vi "PH_uOPA_DelayController.contents.vi"   [LabVIEW 2014, in "PH_uOPA_DelayController.lvlib"]
doc: "This class is forseen to collect andf indicate the measured laser backreflection data.\n\nThis class is part of the PHELIX device layer."
uses:
  PH_uOPA_DelayController.lvlib
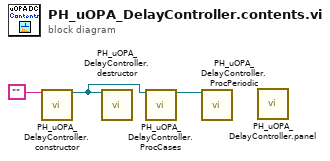
[diagram p0: block diagram]
diagram:
  n1 = call "PH_uOPA_DelayController.constructor.vi"("name"="") -> ("i ref out"=w1:refnum<vi>)  [unwired: 16 in, 2 out]
  n2 = call "PH_uOPA_DelayController.destructor.vi"("i ref in"=w1) -> ()  [unwired: 18 in, 1 out]
  n3 = call "PH_uOPA_DelayController.ProcCases.vi"("i ref in"=w1) -> ("i ref out"=w2:refnum<vi>)  [unwired: 16 in, 2 out]
  n4 = call "PH_uOPA_DelayController.ProcPeriodic.vi"("i ref in"=w2) -> ()  [unwired: 16 in, 3 out]
  n5 = call "PH_uOPA_DelayController.panel.vi"() -> ()  [unwired: 19 in, 1 out]
